vi "Update Status Msg.vi"(8 "error in (no error)":errorcluster, 10 "Ready...":string, 11 "Queue in":refnum<queue>) -> (0 "error out":errorcluster)   [LabVIEW 2018, in "Message Queue.lvlib"]
uses:
  Message Queue.lvlib
  Message Cluster.ctl
  Enqueue Message (Single).vi
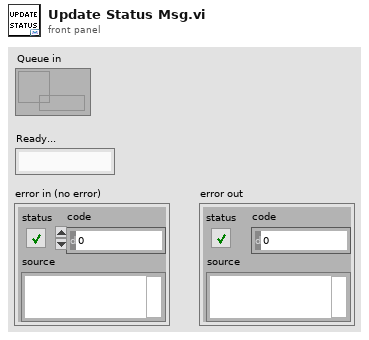
[diagram p1: front panel]
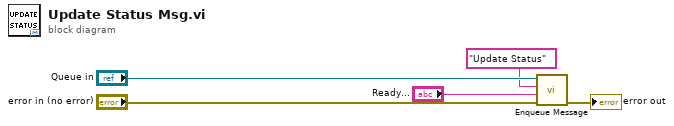
[diagram p0: block diagram]
diagram:
  n1 = call-poly "Enqueue Message.vi"("error in (no error)"="error in (no error)", "Message Data"="Ready...", "Message"="Update Status", "Message Queue"="Queue in") -> ("error out"=→"error out":errorcluster)  [unwired: 6 in, 1 out]
